vi "MVC OOP Advanced with Commands and Factory.vi"() -> ()   [LabVIEW 2011]
doc: "This VI is a basic function generator utilising a class to encapsulate the frequency, type and resulatnt waveform. It also utilises the command pattern design pattern to control the program flow."
uses:
  Advanced Waveform Class/Advanced Waveform.lvclass
  Message Class/Message.lvclass
  Message Class/Initialise Message/Initialise.lvclass
  Message Class/Stop Message/Stop Message.lvclass
  Message Class/Set Frequency Message/Set Frequency Message.lvclass
  Message Class/Generate From File Message/Generate From File.lvclass
  Message Class/FFT Signal Message/FFT Signal Message.lvclass
panel:
  in  "Gen Signal From File":bool
  in  "Waveform from File":i32(ring) items=["Gen Sine.lvclass", "Gen Square.lvclass", "Gen Triangle.lvclass"]
  in  "FFT Signal":bool
  in  "Frequency":dbl(knob) scale=0.0..11.0
  out "Waveform Graph":waveform(dbl)(graph)
  in  "stop":bool
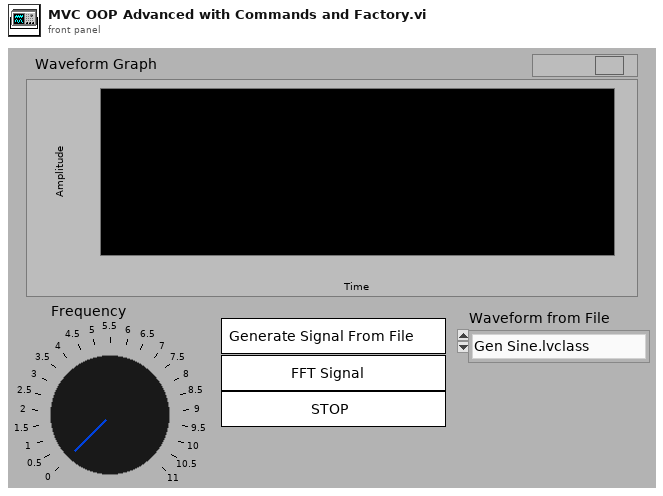
[diagram p1: front panel]
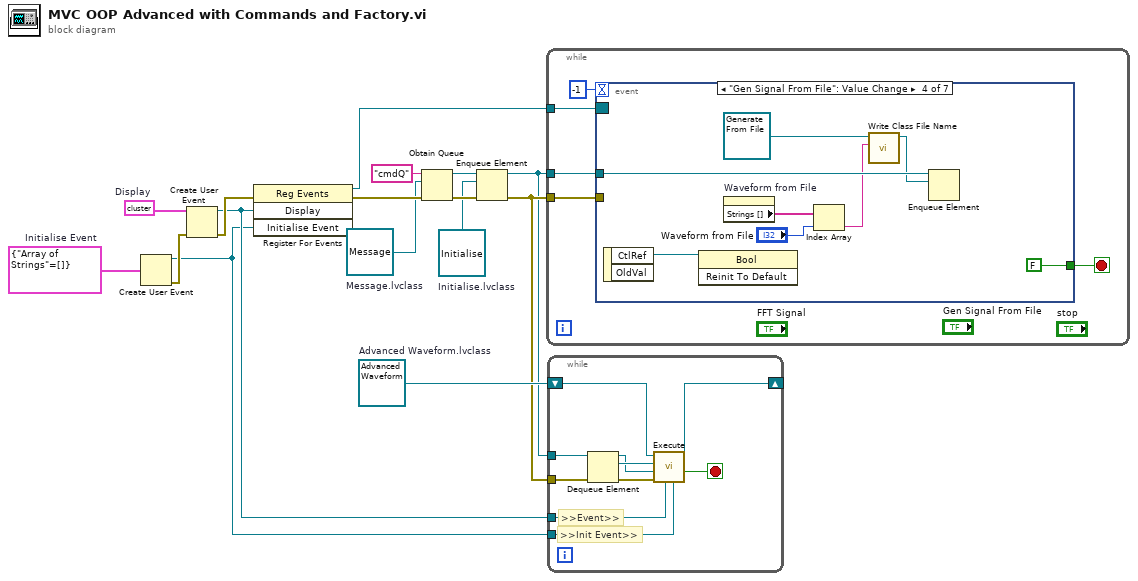
[diagram p0: block diagram]
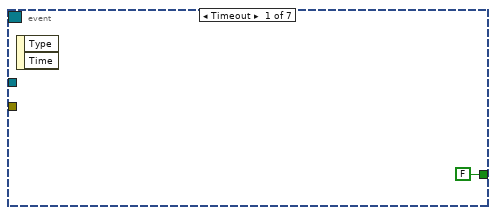
[diagram p2: hidden frame]
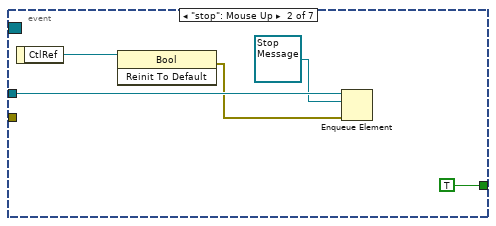
[diagram p3: hidden frame]
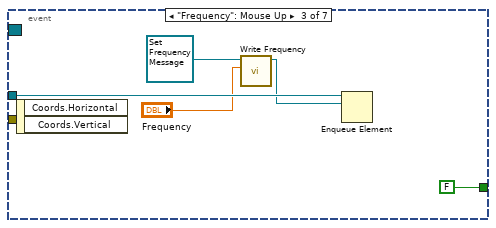
[diagram p4: hidden frame]
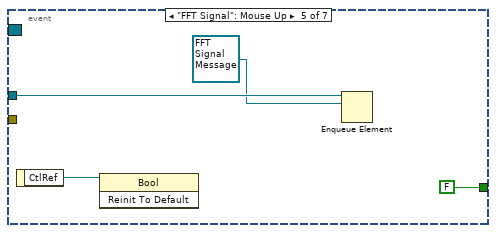
[diagram p5: hidden frame]
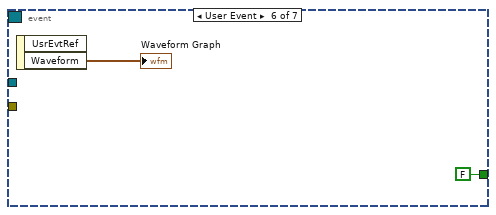
[diagram p6: hidden frame]
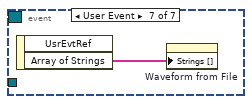
[diagram p7: hidden frame]
diagram:
  w1 = refnum<class "Initialise.lvclass"> refnum  # Initialise.lvclass
  w8 = cluster{"Array of Strings":string[]} {"Array of Strings"=[]}  # Initialise Event
  w9 = refnum<class "Message.lvclass"> refnum  # Message.lvclass
  w10 = refnum<class "Advanced Waveform.lvclass"> refnum  # Advanced Waveform.lvclass
  w14 = cluster{"Waveform":waveform(dbl)} {"Waveform"={"t0"=timestamp(0 s since 1904-01-01), "dt"=1.0, "Y"=[]}}  # Display
  n1 = Create User Event(user event datatype=w8) -> (user event=w6:refnum<user-event>, error out=w7:errorcluster)  [unwired: 1 in]
  n2 = Create User Event(user event datatype=w14, error in=w7) -> (user event=w11:refnum<user-event>, error out=w13:errorcluster)
  n3 = register-events(error in=w13, w11, w6) -> (reference out=w12:refnum<event-registration>, error out=w15:errorcluster)  [unwired: 1 in]
  n4 = Obtain Queue(name (unnamed)="cmdQ", element data type=w9, error in (no error)=w15) -> (queue out=w2:refnum<queue>, error out=w5:errorcluster)  [unwired: 2 in, 1 out]
  n5 = Enqueue Element(queue=w2, element=w1, error in (no error)=w5) -> (queue out=w3:refnum<queue>, error out=w4:errorcluster)  [unwired: 1 in, 1 out]
  n6 = while {
    tunnel: w3 -> [w20]
    tunnel: w12 -> [w18]
    tunnel: w4 -> [w17]
    stop <- w19 stop-if-true
    n7 = event shown="[3] \"Gen Signal From File\": Value Change" {
      selector: w18 -> [_ _ _ _ _ _ _]
      dyn-events: _ -> [_ _ _ _ _ _ _]
      timeout: -1 -> [_ _ _ _ _ _ _]
      tunnel: w20 -> [_ w26 w32 w40 w44 _ _]
      tunnel: [FALSE TRUE FALSE FALSE FALSE FALSE _] -> w19
      tunnel: w17 -> [_ _ _ _ _ _ _]
      event Timeout {
        n8 = event-data() -> ()  [unwired: 1 in, 2 out]
      }
      event "stop": Mouse Up {
        n9 = event-data() -> ("CtlRef"=w27:refnum<vi>)  [unwired: 1 in]
        n10 = invoke class="Bool" method="Reinit To Default"(reference=w27) -> (error out=w25:errorcluster)  [unwired: 2 in, 2 out]
        n11 = Enqueue Element(queue=w26, element=refnum<class "Stop Message.lvclass"> refnum ("Stop Message.lvclass"), error in (no error)=w25) -> ()  [unwired: 1 in, 3 out]
      }
      event "Frequency": Mouse Up {
        n12 = event-data() -> ()  [unwired: 1 in, 2 out]
        n13 = call-dynamic "Write Frequency.vi"("Frequency"="Frequency", "Set Frequency Message in"=refnum<class "Set Frequency Message.lvclass"> refnum ("Set Frequency Message.lvclass")) -> ("Set Frequency Message out"=w28:refnum<class "Set Frequency Message.lvclass">)  [unwired: 8 in, 1 out]
        n14 = Enqueue Element(queue=w32, element=w28) -> ()  [unwired: 2 in, 3 out]
      }
      event "Gen Signal From File": Value Change {
        n15 = event-data() -> ("CtlRef"=w38:refnum<vi>)  [unwired: 1 in, 1 out]
        n16 = invoke class="Bool" method="Reinit To Default"(reference=w38) -> ()  [unwired: 2 in, 3 out]
        n17 = property on="Waveform from File" class="Ring (strict)"() -> ("Strings []"=w37:string[])  [unwired: 2 in, 2 out]
        n18 = Index Array(array=w37, index="Waveform from File") -> (element=w34:string)
        n19 = call-dynamic "Write Class File Name.vi"("Class File Name"=w34, "Generate From File in"=refnum<class "Generate From File.lvclass"> refnum ("Generate From File.lvclass")) -> ("Generate From File out"=w35:refnum<class "Generate From File.lvclass">)  [unwired: 8 in, 1 out]
        n20 = Enqueue Element(queue=w40, element=w35) -> ()  [unwired: 2 in, 3 out]
      }
      event "FFT Signal": Mouse Up {
        n21 = event-data() -> ("CtlRef"=w42:refnum<vi>)  [unwired: 1 in]
        n22 = invoke class="Bool" method="Reinit To Default"(reference=w42) -> ()  [unwired: 2 in, 3 out]
        n23 = Enqueue Element(queue=w44, element=refnum<class "FFT Signal Message.lvclass"> refnum ("FFT Signal Message.lvclass")) -> ()  [unwired: 2 in, 3 out]
      }
      event User Event {
        n24 = event-data() -> ("Waveform"=→"Waveform Graph":waveform(dbl))  [unwired: 1 in, 1 out]
      }
      event User Event {
        n25 = event-data() -> ("Array of Strings"=w47:string[])  [unwired: 1 in, 1 out]
        n26 = property on="Waveform from File" class="Ring (strict)"("Strings []"=w47) -> ()  [unwired: 2 in, 2 out]
      }
    }
  }
  n27 = while {
    tunnel: w4 -> [w56]
    tunnel: w3 -> [w57]
    tunnel: w11 -> [w51]
    shift-right: [w49] -> _
    shift-left: w10 -> [w54]
    tunnel: w6 -> [w48]
    stop <- w50 stop-if-true
    # ">>Init Event>>"
    # ">>Event>>"
    n28 = Dequeue Element(queue=w57, error in (no error)=w56) -> (queue out=w52:refnum<queue>, element=w55:refnum<class "Message.lvclass">, error out=w53:errorcluster)  [unwired: 1 in, 1 out]
    n29 = call-dynamic "Execute.vi"("Init user event out"=w48, "user event in"=w51, "Advanced Waveform In"=w54, "Message in"=w55, "Command Queue"=w52, "error in (no error)"=w53) -> ("Advanced Waveform Out"=w49:refnum<class "Advanced Waveform.lvclass">, "Stop"=w50:bool)  [unwired: 2 in, 2 out]
  }
